vi "Get Test Path By Tag.vi"(4 "TestApplicationContext":refnum<vi>, 6 "TestMethods":path[](array[path]), 7 "Method (testMethod)":enum16{"setUp", "testMethod", "tearDown"}(ring)=enum."testMethod", 8 "error in":errorcluster, 9 "TestProjectClasses":path[](array[path]), 10 "TestMethod Tag":string, 11 "Test Project":path) -> (0 "error out":errorcluster, 2 "Path":path, 3 "TestMethod":string, 5 "TestCase":string)   [LabVIEW 2011, in "GraphicalTestRunner.lvlib"]
uses:
  GraphicalTestRunner.lvlib
  <userlib>/_OpenG.lib/file/file.llb/Strip Path Extension - String__ogtk.vi
  <userlib>/_OpenG.lib/file/file.llb/Strip Path - Arrays__ogtk.vi
  <userlib>/_OpenG.lib/file/file.llb/Strip Path Extension - 1D Array of Strings__ogtk.vi
  <userlib>/_OpenG.lib/file/file.llb/Strip Path - Traditional__ogtk.vi
  <userlib>/_OpenG.lib/file/file.llb/Build Path - Traditional__ogtk.vi
  Classes/TestLoader/TestLoader.lvclass
  Libraries/VITesterUtilities.lvlib
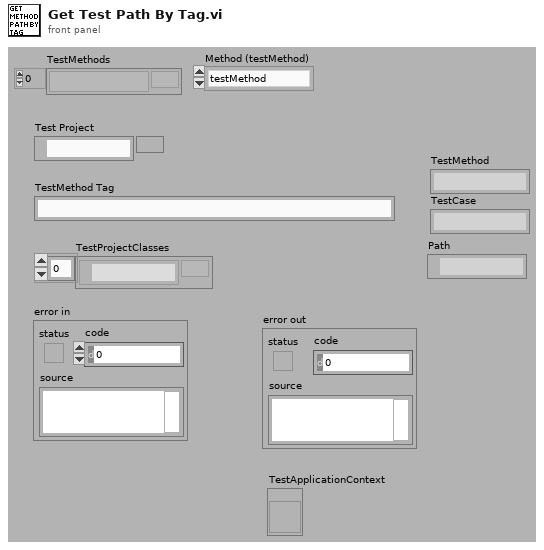
[diagram p1: front panel]
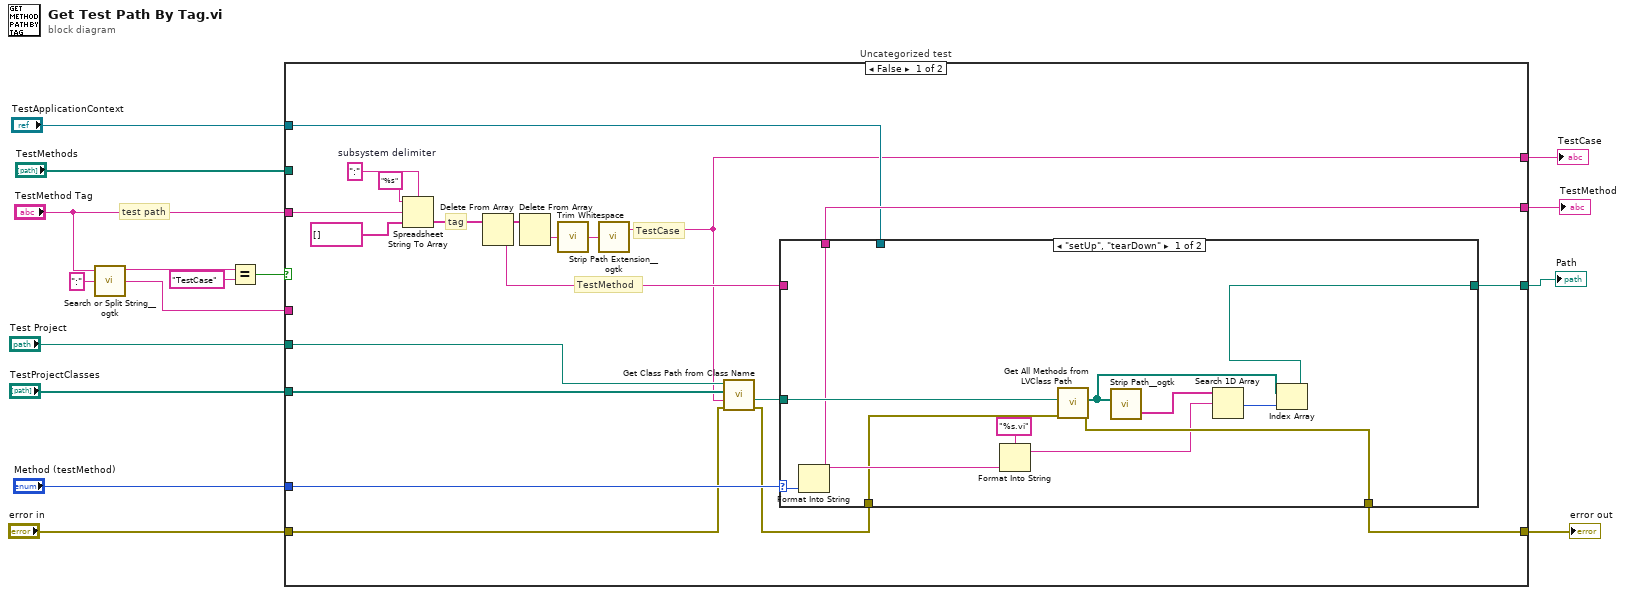
[diagram p0: block diagram]
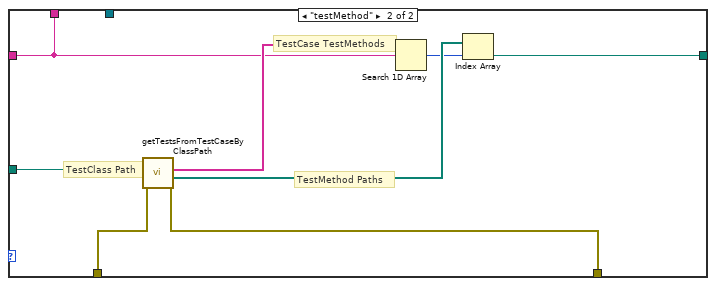
[diagram p2: hidden frame]
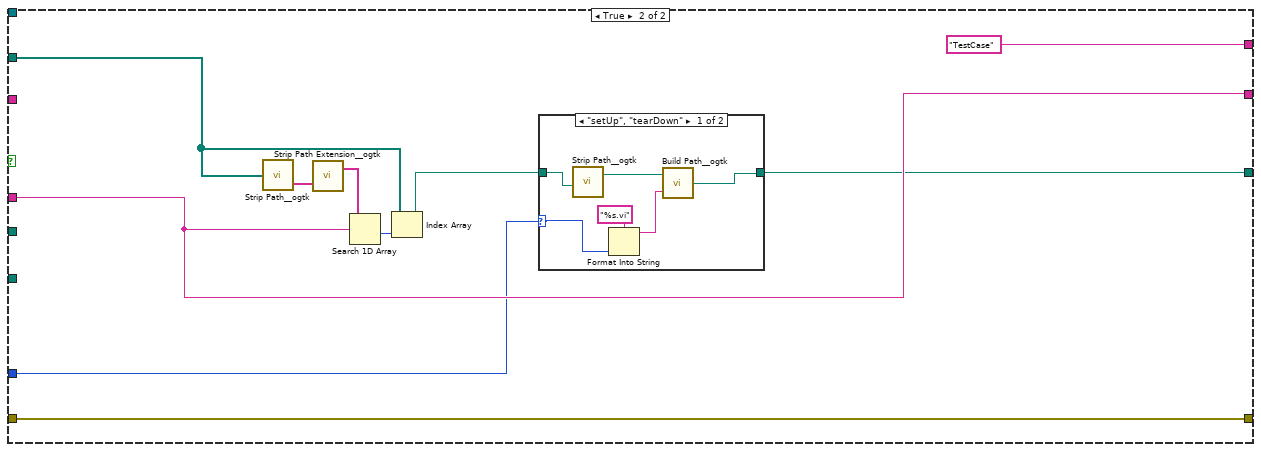
[diagram p3: hidden frame]
diagram:
  # "test path"
  n1 = call <userlib>:"Search or Split String__ogtk.vi"("search string/char (-)"=":", "string"="TestMethod Tag") -> ("substring after match"=w3:string, "substring before match"=w8:string)  [unwired: 1 in, 1 out]
  n2 = Equal?(x=w8, y="TestCase") -> (x = y?=w5:bool)
  n3 = case "Uncategorized test" shown="False" w5 {
    tunnel: [w23 w59] -> w16
    tunnel: [w17 "TestCase"] -> w15
    tunnel: [w30 w61] -> w14
    tunnel: "error in" -> [w20 w61]
    tunnel: [w29 w56] -> w12
    tunnel: "TestProjectClasses" -> [w28 _]
    tunnel: "Test Project" -> [w27 _]
    tunnel: "TestMethod Tag" -> [w26 _]
    tunnel: "TestMethods" -> [_ w62]
    tunnel: w3 -> [_ w59]
    tunnel: "Method (testMethod)" -> [w22 w58]
    tunnel: "TestApplicationContext" -> [w21 _]
    frame False {
      w33 = ":"  # subsystem delimiter
      # "tag"
      # "TestMethod"
      # "TestCase"
      n4 = Spreadsheet String To Array(delimiter (Tab)=w33, format string="%s", spreadsheet string=w26, array type (2D Dbl)=string[] [] ("tests")) -> (array=w34:string[])
      n5 = Delete From Array(array=w34) -> (deleted portion=w24:string, array with subset deleted=w35:string[])  [unwired: 2 in]
      n6 = Delete From Array(array=w35) -> (deleted portion=w36:string)  [unwired: 2 in, 1 out]
      n7 = call <vilib>:"Trim Whitespace.vi"("string"=w36) -> ("trimmed string"=w18:string)  [unwired: 1 in]
      n8 = call-poly <userlib>:"Strip Path Extension__ogtk.vi"("path"=w18) -> ("root"=w17:string)  [unwired: 1 out]
      n9 = call "Get Class Path from Class Name.vi"("error in (no error)"=w20, "Class Name"=w17, "TestProjectClasses"=w28, "Test Project"=w27) -> ("error out"=w19:errorcluster, "Class Path"=w25:path)  [unwired: 6 in]
      n10 = case shown="\"setUp\", \"tearDown\"" w22 {
        selector: w22 -> [w42 _]
        tunnel: w24 -> [_ w48]
        tunnel: [w43 w55] -> w30
        tunnel: w19 -> [w44 w54]
        tunnel: [w45 w51] -> w29
        tunnel: w25 -> [w47 w49]
        tunnel: [w46 w48] -> w23
        tunnel: w21 -> [_ _]
        frame "setUp", "tearDown" {
          n11 = Format Into String(w42) -> (resulting string=w46:string)  [unwired: 3 in, 1 out]
          n12 = Format Into String(format string="%s.vi", w46) -> (resulting string=w39:string)  [unwired: 2 in, 1 out]
          n13 = call "Get All Methods from LVClass Path.vi"("error in"=w44, "class path"=w47) -> ("error out"=w43:errorcluster, "Methods"=w37:path[])  [unwired: 8 in]
          n14 = call-poly <userlib>:"Strip Path__ogtk.vi"("path"=w37) -> ("name"=w40:string[])  [unwired: 1 out]
          n15 = Search 1D Array(1D array=w40, element=w39) -> (index of element=w38:i32)  [unwired: 1 in]
          n16 = Index Array(array=w37, index=w38) -> (element=w45:path)
        }
        frame "testMethod" {
          # "TestMethod Paths"
          # "TestCase TestMethods"
          # "TestClass Path"
          n17 = call "getTestsFromTestCaseByClassPath.vi"("error in"=w54, "TestCase Path"=w49) -> ("error out"=w55:errorcluster, "test paths"=w53:path[], "tests"=w52:string[])  [unwired: 7 in]
          n18 = Search 1D Array(1D array=w52, element=w48) -> (index of element=w50:i32)  [unwired: 1 in]
          n19 = Index Array(array=w53, index=w50) -> (element=w51:path)
        }
      }
    }
    frame True {
      n20 = call-poly <userlib>:"Strip Path__ogtk.vi"("path"=w62) -> ("name"=w63:string[])  [unwired: 1 out]
      n21 = call-poly <userlib>:"Strip Path Extension__ogtk.vi"("paths"=w63) -> ("roots"=w64:string[])  [unwired: 1 out]
      n22 = Search 1D Array(1D array=w64, element=w59) -> (index of element=w65:i32)  [unwired: 1 in]
      n23 = Index Array(array=w62, index=w65) -> (element=w57:path)
      n24 = case shown="\"setUp\", \"tearDown\"" w58 {
        selector: w58 -> [w68 _]
        tunnel: w57 -> [w71 w72]
        tunnel: [w69 w72] -> w56
        frame "setUp", "tearDown" {
          n25 = call-poly <userlib>:"Strip Path__ogtk.vi"("path"=w71) -> ("stripped path"=w70:path)  [unwired: 1 out]
          n26 = Format Into String(format string="%s.vi", w68) -> (resulting string=w66:string)  [unwired: 2 in, 1 out]
          n27 = call-poly <userlib>:"Build Path__ogtk.vi"("name or relative path"=w66, "base path"=w70) -> ("appended path"=w69:path)
        }
        frame "testMethod" {
        }
      }
    }
  }
  "error out" <- w14
  "Path" <- w12
  "TestMethod" <- w16
  "TestCase" <- w15
